vi "Command Sequencer.vi"(6 "Iteration":i32=255, 8 "Command Sequencer Info":T1(array[cluster])) -> ()   [LabVIEW 2019]
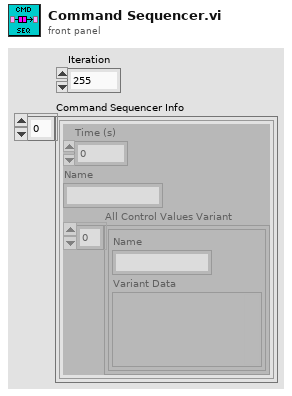
[diagram p1: front panel]
types:
  T1 = cluster{"Time (s)":dbl, "Name":string, "All Control Values Variant":cluster{"Name":string, "Variant Data":variant}[]}[]
  T2 = cluster{"Time (s)":dbl, "Name":string, "All Control Values Variant":cluster{"Name":string, "Variant Data":variant}[]}
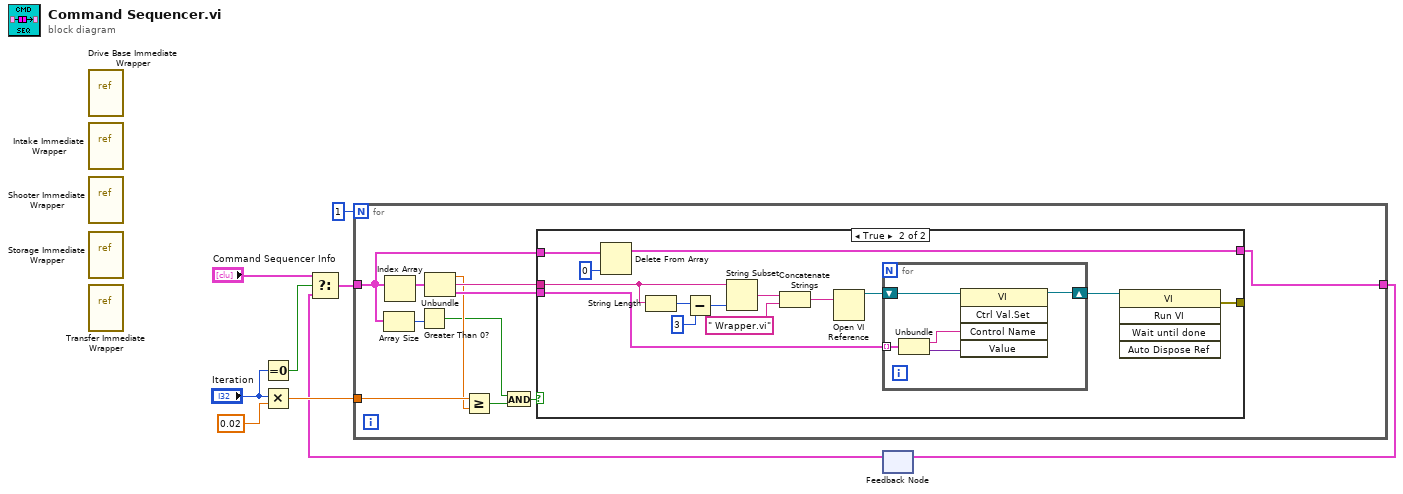
[diagram p0: block diagram]
diagram:
  n1 = vi-ref "Drive Base Immediate Wrapper.vi"() -> ()  [unwired: 1 out]
  n2 = vi-ref "Intake Immediate Wrapper.vi"() -> ()  [unwired: 1 out]
  n3 = vi-ref "Shooter Immediate Wrapper.vi"() -> ()  [unwired: 1 out]
  n4 = vi-ref "Storage Immediate Wrapper.vi"() -> ()  [unwired: 1 out]
  n5 = vi-ref "Transfer Immediate Wrapper.vi"() -> ()  [unwired: 1 out]
  n6 = Equal To 0?(x="Iteration") -> (x = 0?=w5:bool)
  n7 = Multiply(x="Iteration", y=0.02) -> (x*y=w8:dbl)
  n8 = feedback #1() -> (w1:T1)  [unwired: 1 in]
  n9 = Select(t="Command Sequencer Info", s=w5, f=w1) -> (s? t:f=w3:T1)
  n10 = for {
    N: 1 -> [_]
    tunnel: w8 -> [w20]
    tunnel: w3 -> [w14]
    tunnel: [w15] -> w2
    n11 = Array Size(array=w14) -> (size(s)=w11:i32)
    n12 = Index Array(array=w14) -> (element=w16:T2)  [unwired: 1 in]
    n13 = Greater Than 0?(x=w11) -> (x > 0?=w10:bool)
    n14 = Unbundle(w16) -> ("Time (s)"=w17:dbl, "Name"=w19:string, "All Control Values Variant"=w18:cluster{"Name":string, "Variant Data":variant}[])
    n15 = Greater Or Equal?(x=w20, y=w17) -> (x >= y?=w12:bool)
    n16 = And(x=w10, y=w12) -> (x .and. y?=w13:bool)
    n17 = case shown="True" w13 {
      tunnel: w19 -> [_ w35]
      tunnel: w18 -> [_ w27]
      tunnel: w14 -> [w21 w25]
      tunnel: [w21 w24] -> w15
      tunnel: [_ w22] -> _
      frame False {
      }
      frame True {
        n18 = Delete From Array(array=w25, index=0) -> (array with subset deleted=w24:T1)  [unwired: 1 in, 1 out]
        n19 = String Length(string=w35) -> (length=w34:i32)
        n20 = Subtract(x=w34, y=3) -> (x-y=w33:i32)
        n21 = String Subset(string=w35, length (rest)=w33) -> (substring=w31:string)  [unwired: 1 in]
        n22 = Concatenate Strings(w31, " Wrapper.vi" ("string")) -> (w29:string)
        n23 = Open VI Reference(vi path=w29) -> (vi reference=w28:refnum<vi>)  [unwired: 5 in, 1 out]
        n24 = for {
          shift-right: [w39] -> w26
          shift-left: w28 -> [w40]
          tunnel: w27 -> [w38] mode=indexing
          n25 = Unbundle(w38) -> ("Name"=w37:string, "Variant Data"=w36:variant)
          n26 = invoke class="VI" method="Ctrl Val.Set"(reference=w40, "Control Name"=w37, "Value"=w36) -> (reference out=w39:refnum<vi>)  [unwired: 2 in, 4 out]
        }
        n27 = invoke class="VI" method="Run VI"(reference=w26) -> (error out=w22:errorcluster)  [unwired: 4 in, 4 out]
      }
    }
  }
  n28 = feedback-in #1(w2) -> ()
